vi "Introspection Core.vi"(8 "error in (no error)":errorcluster, 11 "Beep in":refnum<class "Beep.lvclass">) -> (0 "error out":errorcluster, 2 "CS++Messages":refnum<class "Message.lvclass">[](array[class]), 3 "Beep out":refnum<class "Beep.lvclass">)   [LabVIEW 2016, in "CS++BeepActor.lvlib" / "Beep.lvclass"]
doc: "This vi delivers a list with all messages this actor reacts to. \n\nNote that all inherited classes have to overwrite it."
uses:
  Beep.lvclass
  <vilib>/ActorFramework/Message/Message.lvclass
  Beep Messages/Beep Msg/Beep Msg.lvclass
  C:/Program Files (x86)/National Instruments/LabVIEW 2016/vi.lib/ActorFramework/Message/Message.lvclass
  Beep Messages/Write Beep Parameters Msg/Write Beep Parameters Msg.lvclass
  CSPP_Core/Actors/CS++BaseActor/CS++BaseActor.lvclass
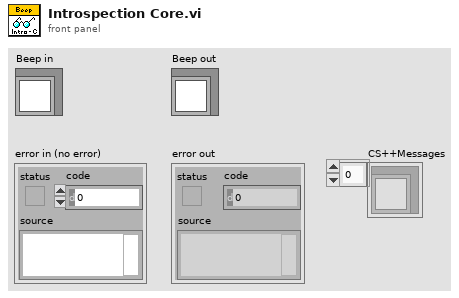
[diagram p1: front panel]
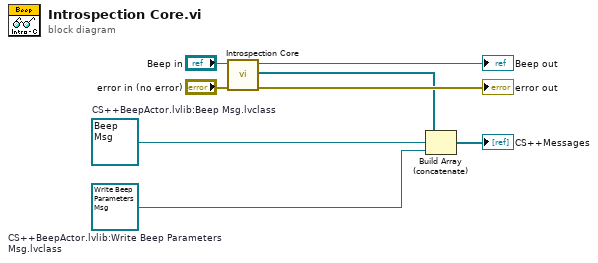
[diagram p0: block diagram]
diagram:
  w1 = refnum<class "Write Beep Parameters Msg.lvclass"> refnum  # CS++BeepActor.lvlib:Write Beep Parameters Msg.lvclass
  w2 = refnum<class "Beep Msg.lvclass"> refnum  # CS++BeepActor.lvlib:Beep Msg.lvclass
  n1 = call-parent "Introspection Core.vi"("error in (no error)"="error in (no error)", "CS++BaseActor in"="Beep in") -> ("error out"=→"error out":errorcluster, "CS++Messages"=w7:refnum<class "Message.lvclass">[], "CS++BaseActor out"=→"Beep out":refnum<class "Beep.lvclass">)  [unwired: 7 in]
  n2 = Build Array (concatenate)(w7, w2, w1) -> (→"CS++Messages":refnum<class "Message.lvclass">[])
